vi "Delete Color Item.vi"(6 "Former Active Slider ID":i32, 8 "error in (no error)":errorcluster, 9 "Numeric Ref Array In":refnum<vi>[](array[refnum]), 10 "Color Ref Array In":refnum<vi>[](array[refnum]), 11 "Slider Ref Array":refnum<vi>[](array[refnum])) -> (0 "error out":errorcluster, 4 "New Active Slider ID":i32)   [LabVIEW 2020, in "3D Plot.lvclass"]
uses:
  <vilib>/Math Plots/3D Math Plots/3D Plot/3D Plot/3D Plot.lvclass
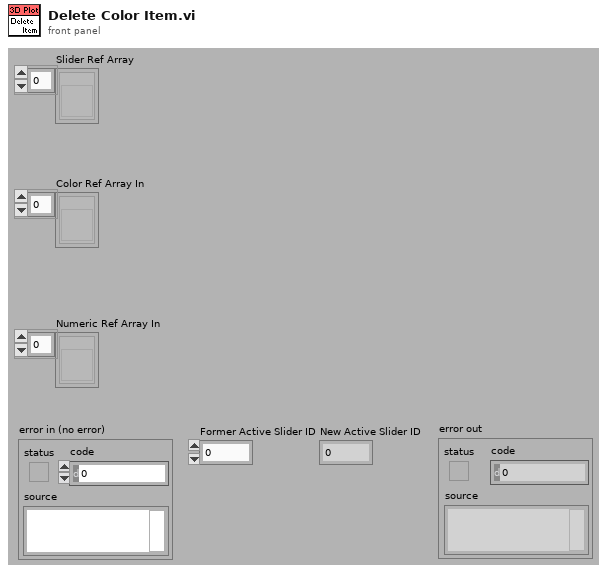
[diagram p1: front panel]
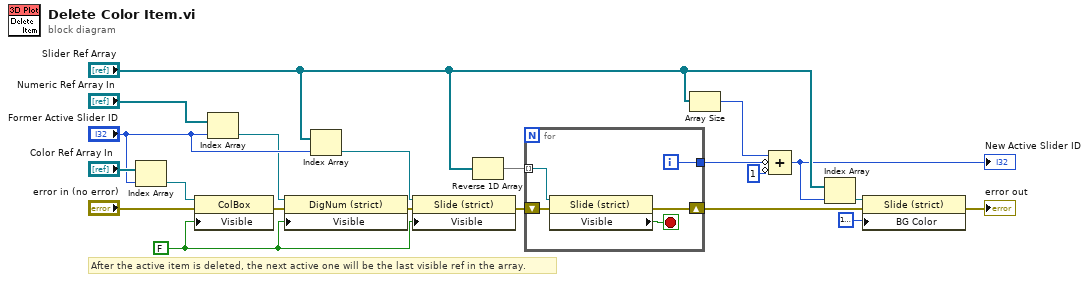
[diagram p0: block diagram]
diagram:
  w15 = FALSE ("Visible")
  # "After the active item is deleted, the next active one will be the last visible ref in the array."
  n1 = Index Array(array="Color Ref Array In", index="Former Active Slider ID") -> (element=w16:refnum<vi>)
  n2 = property class="ColBox"(reference=w16, error in="error in (no error)", "Visible"=w15) -> (error out=w5:errorcluster)  [unwired: 1 out]
  n3 = Index Array(array="Numeric Ref Array In", index="Former Active Slider ID") -> (element=w17:refnum<vi>)
  n4 = property class="DigNum (strict)"(reference=w17, error in=w5, "Visible"=w15) -> (error out=w4:errorcluster)  [unwired: 1 out]
  n5 = Index Array(array="Slider Ref Array", index="Former Active Slider ID") -> (element=w18:refnum<vi>)
  n6 = property class="Slide (strict)"(reference=w18, error in=w4, "Visible"=w15) -> (error out=w3:errorcluster)  [unwired: 1 out]
  n7 = Reverse 1D Array(array="Slider Ref Array") -> (reversed array=w14:refnum<vi>[])
  n8 = for {
    tunnel: w14 -> [w26] mode=indexing
    tunnel: [w24] -> w8
    shift-right: [w22] -> w2
    shift-left: w3 -> [w23]
    i -> [w24]
    stop <- w25 stop-if-true
    n9 = property class="Slide (strict)"(reference=w26, error in=w23) -> (error out=w22:errorcluster, "Visible"=w25:bool)  [unwired: 1 out]
  }
  n10 = Array Size(array="Slider Ref Array") -> (size(s)=w13:i32)
  n11 = Compound Arithmetic op=ADD(w13, invert w8, invert 1 ("value")) -> (w7:i32)
  "New Active Slider ID" <- w7
  n12 = Index Array(array="Slider Ref Array", index=w7) -> (element=w11:refnum<vi>)
  n13 = property class="Slide (strict)"(reference=w11, error in=w2, "BG Color"=u32 16777222) -> (error out=→"error out":errorcluster)  [unwired: 1 out]
